vi "Command Loop - Apply Config.vi"(8 "error in":errorcluster, 10 "Data":u8[](array[numeric]), 11 "Queue Refs in":T1) -> (0 "error out":errorcluster, 2 "Response":string, 3 "Queue Refs out":T1)   [LabVIEW 2025, in "Runtime Configuration Support Inline Async Example Engine.lvlib"]
uses:
  Runtime Configuration Support Inline Async Example Engine.lvlib
  Shared/ReConfigured.Settings.ctl
  Shared/Compiled.Settings.ctl
  <vilib>/NI VeriStand/Custom Device API/Block Data Reference.ctl
  <vilib>/NI VeriStand/Custom Device API/Data Reference.ctl
  <vilib>/NI VeriStand/Custom Device API/Custom Device API.lvlib
  Shared/Runtime Configuration Support Inline Async Example Shared.lvlib
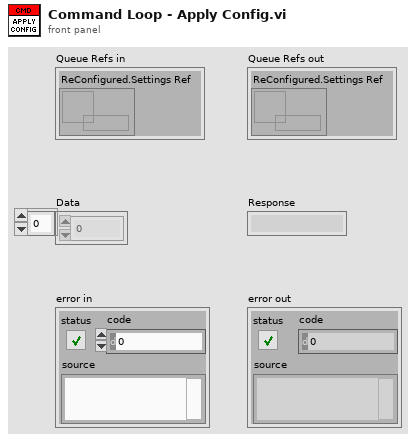
[diagram p1: front panel]
types:
  T1 = cluster{"ReConfigured.Settings Ref":refnum<queue>}
  T2 = cluster{"Dynamic Config Status":bool, "Error":errorcluster}
  T3 = typedef "Runtime Configuration Support Inline Async Example Shared.lvlib/ReConfigured.Settings.ctl" = cluster{"Compiled.Settings":T4, "Compiled Inline Async Settings":cluster{"Read":cluster{"Refs":T5[], "Values":dbl[]}[], "Write":cluster{"Refs":T5[], "Values":dbl[]}[], "ReadWrite":cluster{"Refs":T6[], "Values":dbl[], "Reset Values":dbl[]}[], "LUT":variant}, "Response Ref":refnum<queue>}
  T4 = typedef "Runtime Configuration Support Inline Async Example Shared.lvlib/Compiled.Settings.ctl" = cluster{"Name":string, "Async Init Timeout":u16, "Inport SignalIDs":i32[], "Outport SignalIDs":i32[], "Inport Values":dbl[], "Outport Values":dbl[], "Dynamic Config Status":bool, "Device Error":errorcluster}
  T5 = typedef "Custom Device API.lvlib/Block Data Reference.ctl" = cluster{"Data Reference":T6, "Offset":u64, "Length":u64}
  T6 = typedef "Custom Device API.lvlib/Data Reference.ctl" = i32
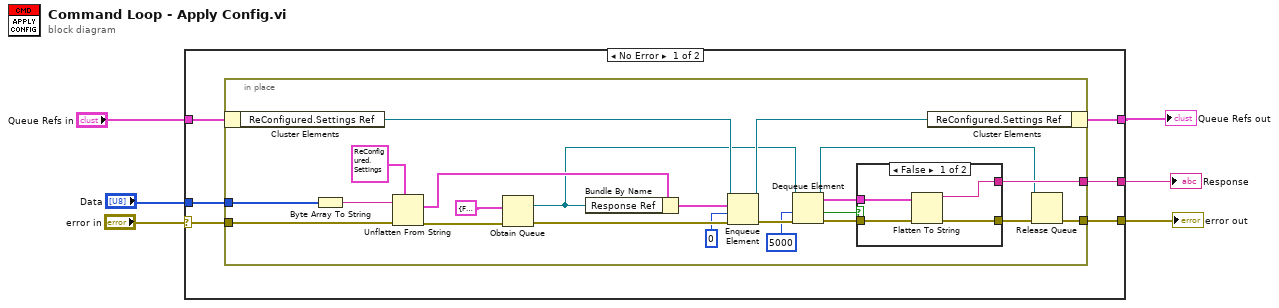
[diagram p0: block diagram]
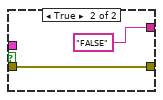
[diagram p2: hidden frame]
diagram:
  n1 = case shown="No Error" "error in" {
    selector: "error in" -> [w11 w42]
    tunnel: [w12 w42] -> w6
    tunnel: "Data" -> [w10 _]
    tunnel: [w9 _] -> w3
    tunnel: "Queue Refs in" -> [w8 w41]
    tunnel: [w7 w41] -> w1
    frame No Error {
      n2 = in-place {
        in-place-border: [w30] -> w12
        in-place-border: w11 -> [w32]
        in-place-border: w10 -> [w26]
        in-place-border: [w25] -> w9
        n3 = in-place-cluster #1(w8) -> ("ReConfigured.Settings Ref"=w23:refnum<queue>)
        n4 = Byte Array To String(unsigned byte array=w26) -> (string=w27:string)
        n5 = Unflatten From String(type=T3 {"Compiled.Settings"={"Name"="", "Async Init Timeout"=0, "Inport SignalIDs"=[], "Outport SignalIDs"=[], "Inport Values"=[], "Outport Values"=[], "Dynamic Config Status"=FALSE, "Device Error"={"status"=FALSE, "code"=0, "source"=""}}, "Compiled Inline Async Settings"={"Read"=[], "Write"=[], "ReadWrite"=[], "LUT"=variant}, "Response Ref"=refnum} ("ReConfigured.Settings"), binary string=w27, error in (no error)=w32) -> (value=w21:T3, error out=w34:errorcluster)  [unwired: 2 in, 1 out]
        n6 = Obtain Queue(element data type=T2 {"Dynamic Config Status"=FALSE, "Error"={"status"=FALSE, "code"=0, "source"=""}}, error in (no error)=w34) -> (queue out=w16:refnum<queue>, error out=w33:errorcluster)  [unwired: 3 in, 1 out]
        n7 = Bundle By Name(cluster=w21, "Response Ref"=w16) -> (w14:T3)
        n8 = Enqueue Element(queue=w23, element=w14, timeout in ms (-1)=0, error in (no error)=w33) -> (queue out=w22:refnum<queue>, error out=w31:errorcluster)  [unwired: 1 out]
        n9 = Dequeue Element(queue=w16, timeout in ms (-1)=5000, error in (no error)=w31) -> (queue out=w17:refnum<queue>, element=w20:T2, timed out?=w19:bool, error out=w28:errorcluster)
        n10 = case shown="False" w19 {
          tunnel: w20 -> [w35 _]
          tunnel: [w36 "FALSE"] -> w25
          tunnel: w28 -> [w38 w40]
          tunnel: [w37 w40] -> w29
          frame False {
            n11 = Flatten To String(anything=w35, error in (no error)=w38) -> (data string=w36:string, error out=w37:errorcluster)  [unwired: 2 in, 1 out]
          }
          frame True {
          }
        }
        n12 = in-place-cluster #1("ReConfigured.Settings Ref"=w22) -> (w7:T1)
        n13 = Release Queue(queue=w17, error in (no error)=w29) -> (error out=w30:errorcluster)  [unwired: 1 in, 2 out]
      }
    }
    frame Error {
    }
  }
  "error out" <- w6
  "Response" <- w3
  "Queue Refs out" <- w1
